vi "cursors.vi"(10 "X1 (s)":dbl, 11 "XYGraph in":refnum<vi>) -> (3 "Cluster":cluster{dbl[], dbl[]})   [LabVIEW 2021]
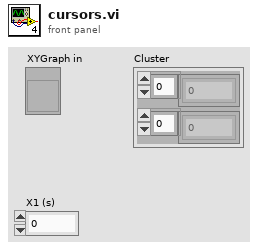
[diagram p1: front panel]
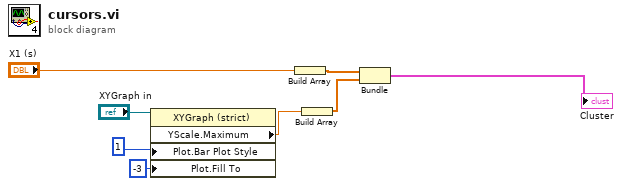
[diagram p0: block diagram]
diagram:
  n1 = property on="Property Node" class="XYGraph (strict)"(reference="XYGraph in", "Plot.Bar Plot Style"=u8 1, "Plot.Fill To"=i16 -3) -> ("YScale.Maximum"=w5:dbl)  [unwired: 1 in, 2 out]
  n2 = Build Array("X1 (s)") -> (w2:dbl[])
  n3 = Build Array(w5) -> (w3:dbl[])
  n4 = Bundle(w2, w3) -> (→"Cluster":cluster{dbl[], dbl[]})  [unwired: 1 in]
